vi "2-Stopwatch.vi"() -> ()   [LabVIEW 2014]
panel:
  out "Eslapsed Time (seconds)":dbl format="%#.2g"
  in  "Stop Button":bool
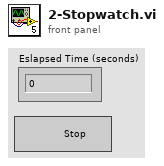
[diagram p1: front panel]
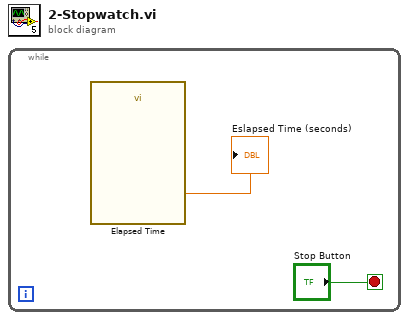
[diagram p0: block diagram]
diagram:
  n1 = while {
    stop <- "Stop Button" stop-if-true
    n2 = call "Elapsed Time"() -> ("Elapsed Time (s)"=→"Eslapsed Time (seconds)":dbl)  [unwired: 12 in, 7 out]
  }
